vi "Develop Tools - ScratchRename.vi"   [LabVIEW 2011]
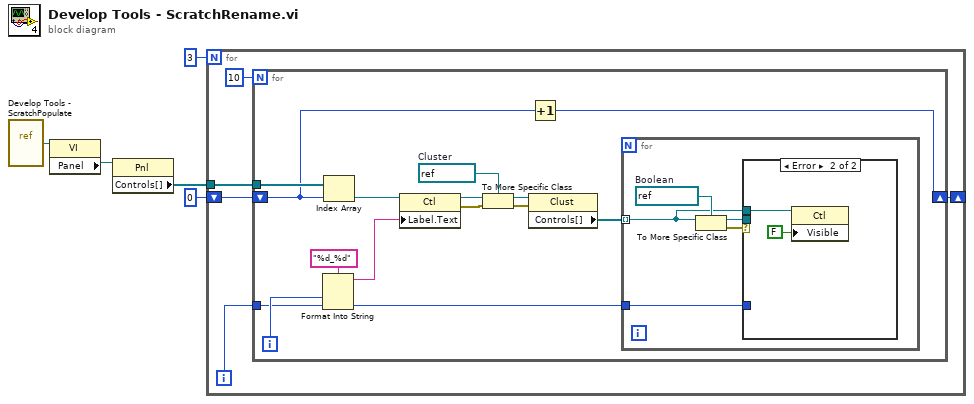
[diagram p0: block diagram]
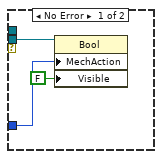
[diagram p2: hidden frame]
diagram:
  n1 = vi-ref "Develop Tools - ScratchPopulate.vi"() -> (w5:refnum<vi>)
  n2 = property class="VI"(reference=w5) -> ("Panel"=w4:refnum<vi>)  [unwired: 1 in, 2 out]
  n3 = property class="Pnl"(reference=w4) -> ("Controls[]"=w2:refnum<vi>[])  [unwired: 1 in, 2 out]
  n4 = for {
    N: 3 -> [_]
    tunnel: w2 -> [w9]
    shift-right: [w7] -> _
    shift-left: 0 -> [w8]
    i -> [w6]
    n5 = for {
      N: 10 -> [_]
      tunnel: w9 -> [w23]
      tunnel: w6 -> [w17]
      shift-right: [w21] -> w7
      shift-left: w8 -> [w22]
      i -> [w18]
      w14 = refnum<vi> refnum  # Cluster
      n6 = Format Into String(format string="%d_%d", w18, w17) -> (resulting string=w19:string)  [unwired: 2 in, 1 out]
      n7 = Index Array(array=w23, index=w22) -> (element=w20:refnum<vi>)
      n8 = property class="Ctl"(reference=w20, "Label.Text"=w19) -> (reference out=w16:refnum<vi>, error out=w15:errorcluster)  [unwired: 1 in]
      n9 = To More Specific Class(target class=w14, reference=w16, error in=w15) -> (specific class reference=w13:refnum<vi>, error out=w12:errorcluster)
      n10 = property class="Clust"(reference=w13, error in=w12) -> ("Controls[]"=w11:refnum<vi>[])  [unwired: 2 out]
      n11 = Increment(x=w22) -> (x+1=w21:i32)
      n12 = for {
        tunnel: w17 -> [w26]
        tunnel: w11 -> [w25] mode=indexing
        w29 = refnum<vi> refnum  # Boolean
        n13 = To More Specific Class(target class=w29, reference=w25) -> (specific class reference=w27:refnum<vi>, error out=w28:errorcluster)  [unwired: 1 in]
        n14 = case shown="Error" w28 {
          tunnel: w27 -> [w32 _]
          tunnel: w26 -> [w31 _]
          tunnel: w25 -> [_ w34]
          frame No Error {
            n15 = property class="Bool"(reference=w32, "MechAction"=w31, "Visible"=FALSE) -> ()  [unwired: 1 in, 2 out]
          }
          frame Error {
            n16 = property class="Ctl"(reference=w34, "Visible"=FALSE) -> ()  [unwired: 1 in, 2 out]
          }
        }
      }
    }
  }
